vi "Write Configuration Version.vi"(8 "error in (no error)":errorcluster, 10 "Configuration Version":T1, 11 "refnum":T2) -> (0 "error out":errorcluster, 3 "refnum out":T2)   [LabVIEW 2017, in "DSF Configuration API.lvlib"]
doc: "Writes a value to a key in a specified section of the configuration data identified by <B>refnum</B>. This VI modifies data in memory. To write data to disk, use the Close Config Data VI. Wire data to the <B>value</B> input to determine the polymorphic instance to use or manually select the instance."
uses:
  DSF Configuration API.lvlib
  Public/Controls/DSF Config Data RefNum.ctl
  Public/Controls/Version Info.ctl
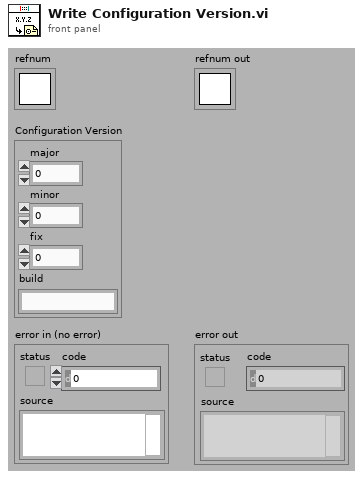
[diagram p1: front panel]
types:
  T1 = typedef "DSF Configuration API.lvlib/Version Info.ctl" = cluster{"major":u32, "minor":u32, "fix":u32, "build":string}
  T2 = typedef "DSF Configuration API.lvlib/DSF Config Data RefNum.ctl" = refnum<k1>
  T3 = typedef "DSF Configuration API.lvlib/Config Queue.ctl" = refnum<queue>
  T4 = typedef "DSF Configuration API.lvlib/Config Data.ctl" = cluster{"dsf configuration":T5, "path":path, "dirty":bool}
  T5 = typedef "DSF Configuration API.lvlib/DSF Config.ctl" = cluster{"dsfversion":T1, "version":T1, "plugins":T6[], "groups":T9[], "transfers":T11[], "channels":T13[], "settings":T15[]}
  T6 = typedef "DSF Configuration API.lvlib/DSF Plugin.ctl" = cluster{"id":string, "values":T7}
  T7 = typedef "DSF Configuration API.lvlib/DSF Plugin Info.ctl" = cluster{"type":string, "timing":T8, "group ids":string[], "settings id":string}
  T8 = typedef "DSF Configuration API.lvlib/DSF Timing Info.ctl" = cluster{"decimation":i32, "offset":i32}
  T9 = typedef "DSF Configuration API.lvlib/DSF Group.ctl" = cluster{"id":string, "values":T10}
  T10 = typedef "DSF Configuration API.lvlib/DSF Group Info.ctl" = cluster{"direction":i32, "timing":T8, "transfer ids":string[], "settings id":string}
  T11 = typedef "DSF Configuration API.lvlib/DSF Transfer.ctl" = cluster{"id":string, "values":T12}
  T12 = typedef "DSF Configuration API.lvlib/DSF Transfer Info.ctl" = cluster{"byte order":i32, "channel ids":string[], "settings id":string}
  T13 = typedef "DSF Configuration API.lvlib/DSF Channel.ctl" = cluster{"id":string, "values":T14}
  T14 = typedef "DSF Configuration API.lvlib/DSF Channel Info.ctl" = cluster{"count":i32, "offset":i32, "data type":i32, "resource path":string, "settings id":string}
  T15 = typedef "DSF Configuration API.lvlib/DSF Settings.ctl" = cluster{"id":string, "values":T16}
  T16 = typedef "DSF Configuration API.lvlib/DSF Settings Info.ctl" = cluster{"key":string, "value":string}[]
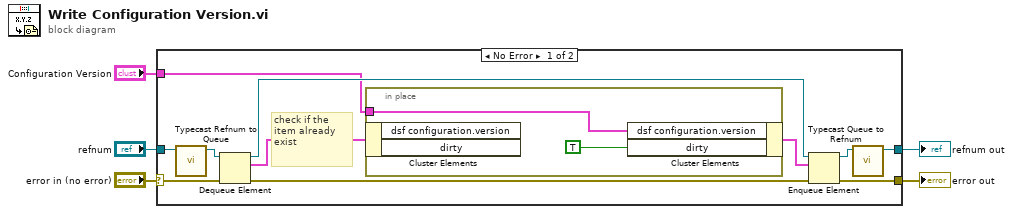
[diagram p0: block diagram]
diagram:
  n1 = case shown="No Error" "error in (no error)" {
    selector: "error in (no error)" -> [w11 w20]
    tunnel: [w15 w20] -> w3
    tunnel: [w13 w19] -> w4
    tunnel: "Configuration Version" -> [w7 _]
    tunnel: "refnum" -> [w6 w19]
    frame No Error {
      # "check if the item already exist"
      n2 = call "Typecast Refnum to Queue.vi"("refnum in"=w6) -> ("queue out"=w12:T3)  [unwired: 10 out]
      n3 = Dequeue Element(queue=w12, error in (no error)=w11) -> (queue out=w16:T3, element=w10:T4, error out=w9:errorcluster)  [unwired: 2 out]
      n4 = in-place {
        in-place-border: w7 -> [w17]
        n5 = in-place-cluster #1(w10) -> ()  [unwired: 2 out]
        n6 = in-place-cluster #1("dsf configuration.version"=w17, "dirty"=TRUE) -> (w8:T4)
      }
      n7 = Enqueue Element(queue=w16, element=w8, error in (no error)=w9) -> (queue out=w14:T3, error out=w15:errorcluster)  [unwired: 2 out]
      n8 = call "Typecast Queue to Refnum.vi"("queue in"=w14) -> ("refnum out"=w13:T2)  [unwired: 10 out]
    }
    frame Error {
    }
  }
  "error out" <- w3
  "refnum out" <- w4
